vi "Send OCP.vi"(8 "error in (no error)":errorcluster, 11 "79XRP in":refnum<class "7976A.lvclass">) -> (0 "error out":errorcluster, 3 "79XRP out":refnum<class "7976A.lvclass">)   [LabVIEW 2019, in "7976A.lvlib" / "7976A.lvclass"]
uses:
  Library/7976A.lvclass
  C:/Users/Public/Documents/Development/builds/Instruments/PowerSupply.lvlibp/Library/PowerSupply.lvclass
  Library/7976A.lvclass/7976A.ctl
  builds/Engine/Engine.lvlibp/Project/Engine.lvclass
  <instrlib>/Agilent N7976A/Agilent N7976A.lvlib
  C:/Users/Public/Documents/Development/builds/Engine/Engine.lvlibp/Project/Engine.lvclass
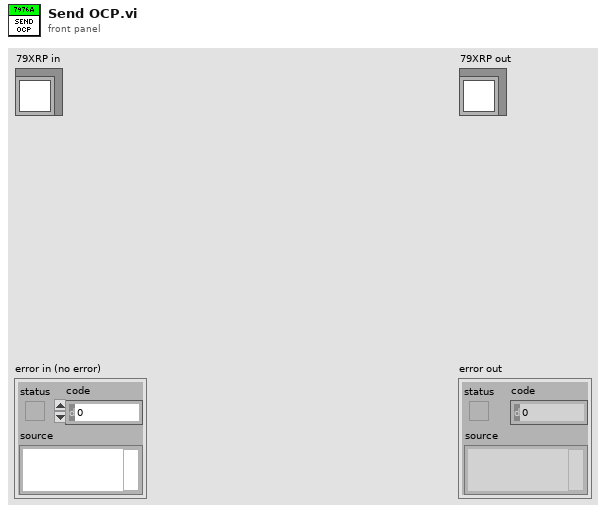
[diagram p1: front panel]
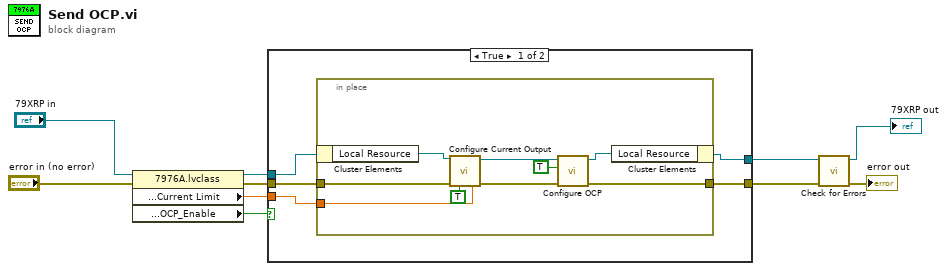
[diagram p0: block diagram]
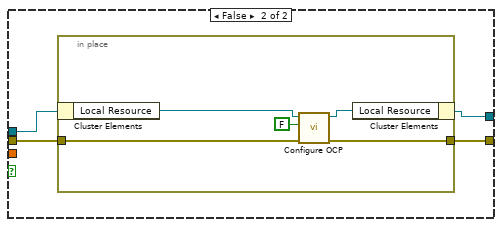
[diagram p2: hidden frame]
diagram:
  n1 = property class="7976A.lvclass"(reference="79XRP in", error in="error in (no error)") -> (reference out=w6:refnum<class "7976A.lvclass">, error out=w5:errorcluster, "Accessors:Setting:Protection:Current Limit"=w2:dbl, "Accessors:Setting:Protection:OCP_Enable"=w1:bool)
  n2 = case shown="True" w1 {
    tunnel: w6 -> [w15 w28]
    tunnel: w5 -> [w14 w27]
    tunnel: [w13 w26] -> w4
    tunnel: [w12 w25] -> w3
    tunnel: w2 -> [w11 _]
    frame True {
      n3 = in-place {
        in-place-border: w14 -> [w24]
        in-place-border: [w17] -> w13
        in-place-border: w11 -> [w22]
        n4 = in-place-cluster #1(w15) -> ("Local Resource"=w23:refnum<visa-resource-name>)
        n5 = call <instrlib>:"Configure Current Output.vi"("VISA resource name"=w23, "error in (no error)"=w24, "Enable Voltage Priority (False)"=TRUE, "Voltage Priority Current Upper Limit (2.50A)"=w22) -> ("VISA resource name out"=w20:refnum<visa-resource-name>, "error out"=w19:errorcluster)  [unwired: 10 in]
        n6 = call <instrlib>:"Configure OCP.vi"("error in (no error)"=w19, "Enable OCP (F: Disabled)"=TRUE, "VISA resource name"=w20) -> ("error out"=w17:errorcluster, "VISA resource name out"=w18:refnum<visa-resource-name>)  [unwired: 7 in]
        n7 = in-place-cluster #1("Local Resource"=w18) -> (w12:refnum<class "7976A.lvclass">)
      }
    }
    frame False {
      n8 = in-place {
        in-place-border: w27 -> [w33]
        in-place-border: [w30] -> w26
        n9 = in-place-cluster #2(w28) -> ("Local Resource"=w32:refnum<visa-resource-name>)
        n10 = call <instrlib>:"Configure OCP.vi"("error in (no error)"=w33, "Enable OCP (F: Disabled)"=FALSE, "VISA resource name"=w32) -> ("error out"=w30:errorcluster, "VISA resource name out"=w31:refnum<visa-resource-name>)  [unwired: 7 in]
        n11 = in-place-cluster #2("Local Resource"=w31) -> (w25:refnum<class "7976A.lvclass">)
      }
    }
  }
  n12 = call "Check for Errors.vi"("error in"=w4, "Engine in"=w3) -> ("error out"=→"error out":errorcluster, "Engine out"=→"79XRP out":refnum<class "7976A.lvclass">)  [unwired: 8 in]
